vi "Packet Read Header.vi"(8 "error in (no error)":errorcluster, 10 "Data":u8[](array[numeric]), 11 "Packet in":refnum<class "Packet.lvclass">) -> (0 "error out":errorcluster, 3 "Packet out":refnum<class "Packet.lvclass">)   [LabVIEW 2019, in "Packet.lvclass"]
uses:
  Packet.lvclass
  Packet.lvclass/Packet.ctl
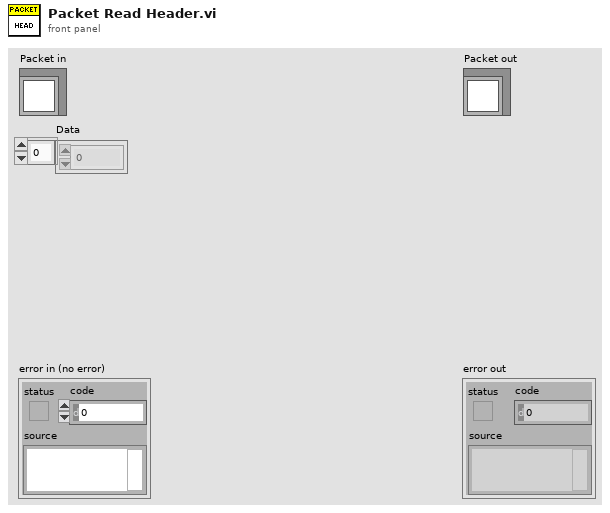
[diagram p1: front panel]
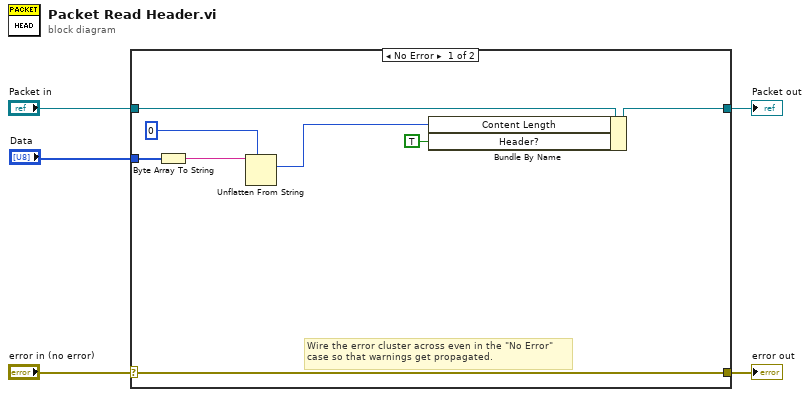
[diagram p0: block diagram]
diagram:
  n1 = case shown="No Error" "error in (no error)" {
    selector: "error in (no error)" -> [w12 w15]
    tunnel: [w12 w15] -> w4
    tunnel: [w8 w14] -> w2
    tunnel: "Packet in" -> [w13 w14]
    tunnel: "Data" -> [w11 _]
    frame No Error {
      # "Wire the error cluster across even in the \"No Error\"\ncase so that warnings get propagated."
      n2 = Byte Array To String(unsigned byte array=w11) -> (string=w10:string)
      n3 = Unflatten From String(type=0, binary string=w10) -> (value=w7:i32)  [unwired: 3 in, 2 out]
      n4 = Bundle By Name(cluster=w13, "Content Length"=w7, "Header?"=TRUE ("Packet Reading Progress.Header?")) -> (w8:refnum<class "Packet.lvclass">)
    }
    frame Error {
    }
  }
  "error out" <- w4
  "Packet out" <- w2
